vi "Drive Controller.vi"(8 "error in":errorcluster) -> ()   [LabVIEW 2019]
doc: "This VI executes continuously carrying out the current operation and responding to updates or new operation requests. It will often contain the timing or control code that is difficult to place directly in TeleOp. This VI generally opens all sensors and motors and isolates the rest of the robot code from knowing implementation details of how the operations are carried out."
uses:
  <vilib>/Rock Robotics/WPI/Framework/Completion Status.ctl
  Drive Setpoints.ctl
  Drive Operations.ctl
  <vilib>/Rock Robotics/WPI/SafetyOutput/WPI_SafetyOutputConfigMenu.ctl
  <vilib>/Rock Robotics/WPI/RobotDrive/WPI_RobotDriveOpen2MotorWithExistingMotors.vi
panel:
  in  "Radio Buttons":enum32{"Outdoor", "Indoor"}(radio)
  in  "Interactive Values":T1
  in  "Buttons":cluster{"Execute Cmd":bool, "Abort Cmd":bool}
  out "Command Timing":cluster{"Start Time (ms)":u32, "Iterations":i32}
  out "Status":T3
  out "Setpoints":T4(graph)
  out "Current\nCmd":string
  # "Tip: The graph shows the motor setpoints. It may also be helpful to observe inputs and sensor values.\nYou may also want to display tuning or debugging controls."
  # "Interactive Command: You may fill in the settings for a command\nand schedule it with the Execute button. You can observe and abort\nany command while fine tuning the code for the controller."
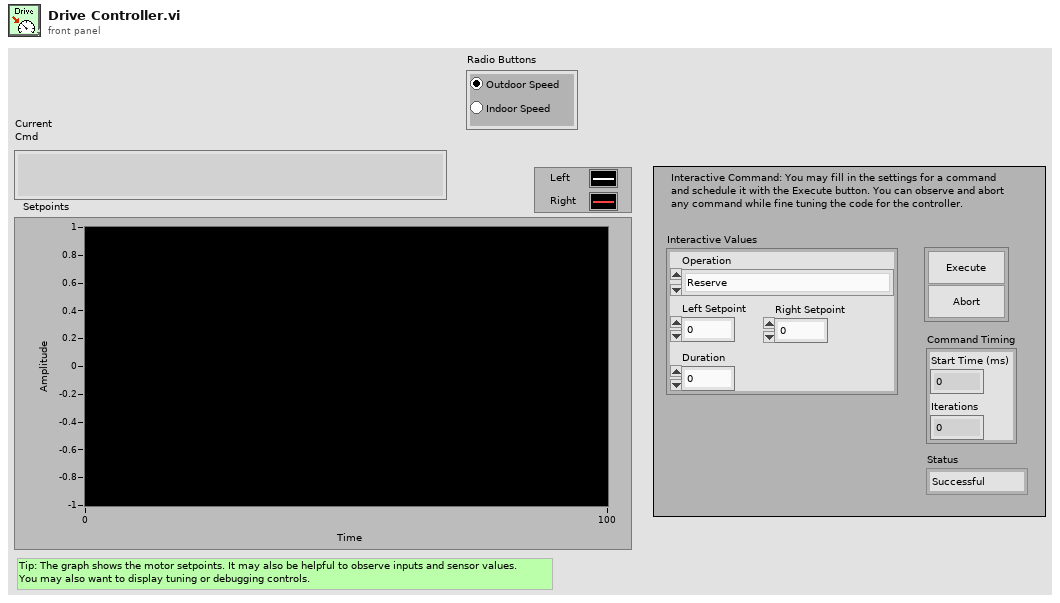
[diagram p1: front panel]
types:
  T1 = typedef "Drive Setpoints.ctl" = cluster{"Operation":T2, "Left Setpoint":dbl, "Right Setpoint":dbl, "Duration":dbl}
  T2 = typedef "Drive Operations.ctl" = enum16{"Reserve", "Read Current", "Immediate", "Drive for Time", "Drive for Distance"}
  T3 = typedef "Completion Status.ctl" = enum16{"Successful", "Aborted", "Incomplete"}
  T4 = cluster{"Left Setpoint":dbl, "Right Setpoint":dbl}
  T5 = enum16{"FollowerType_PercentOutput", "FollowerType_AuxOutput1"}
  T6 = typedef "WPI_SafetyOutputConfigMenu.ctl" = enum16{"Enable", "Disable"}
  T7 = typedef "WPI_MotorControlDeviceRef.ctl" = cluster{"DeviceStatus":errorcluster, "Type":T8, "PWM":cluster{"PWM Channel":T9, "DeadBand":T10}, "CAN":cluster{"Device Number":u8, "SetOutput VI Ref":variant, "GetOutput VI Ref":variant, "Enable VI Ref":variant, "Disable VI Ref":variant, "Data":variant}, "Invert":bool, "DIO PWM":cluster{"PWM \"Enable\" Channel":T9, "DIOChannel":T11, "PWM Rate":dbl}}
  T8 = typedef "WPI_MotorControlType.ctl" = enum16{"PWM", "CAN", "DIO PWM"}
  T9 = typedef "FPGA_DIOPWMChannel.ctl" = enum8{"PWM 0", "PWM 1", "PWM 2", "PWM 3", "PWM 4", "PWM 5", "PWM 6", "PWM 7", "PWM 8", "PWM 9", "PWM MXP 0", "PWM MXP 1", "PWM MXP 2", "PWM MXP 3", "PWM MXP 4", "PWM MXP 5", "PWM MXP 6", "PWM MXP 7", "PWM MXP 8", "PWM MXP 9", "Invalid"}
  T10 = typedef "WPI_PWMDeadband.ctl" = cluster{"Name":string, "maxPositivePwm":i32, "minPositivePwm":i32, "centerPwm":i32, "maxNegativePwm":i32, "minNegativePwm":i32, "angularRange":u16}
  T11 = typedef "FPGA_DIOChannel.ctl" = enum8{"DIO 0", "DIO 1", "DIO 2", "DIO 3", "DIO 4", "DIO 5", "DIO 6", "DIO 7", "DIO 8", "DIO 9", "DIO MXP 0", "DIO MXP 1", "DIO MXP 2", "DIO MXP 3", "DIO MXP 4", "DIO MXP 5", "DIO MXP 6", "DIO MXP 7", "DIO MXP 8", "DIO MXP 9", "DIO MXP 10", "DIO MXP 11", "DIO MXP 12", "DIO MXP 13", "DIO MXP 14", "DIO MXP 15", "SPI Port CS1", "SPI Port CS2", "SPI Port CS3", "SPI Port MISO", "SPI Port MOSI", "Invalid"}
  T12 = typedef "WPI_RobotDriveDevRef.ctl" = cluster{"DevStatus":errorcluster, "Motors[]":T7[], "Square Inputs":bool, "Max Output":dbl}
  T13 = typedef "Command Status Info.ctl" = cluster{"Name":string, "Status":T3, "notifier out":T14}
  T14 = typedef "Completion Notifier.ctl" = refnum<notifier>
  T15 = cluster{"SubSystem Data":T1, cluster{"Start Time (ms)":u32, "Iterations":i32}, cluster{"Command Info":T13, "Description":string, "Default Command":T1, "queue out":refnum<queue>, "Subsystem Name":string}}
  T16 = cluster{"SubSystem Data":T1, cluster{"Start Time (ms)":u32, "Iterations":i32}, "Default Command Arguments":cluster{"Command Info":T13, "Description":string, "Default Command":T1, "queue out":refnum<queue>, "Subsystem Name":string}}
  T17 = cluster{"Don't move motors while reserved":dbl, "Don't move motors while reserved":dbl}
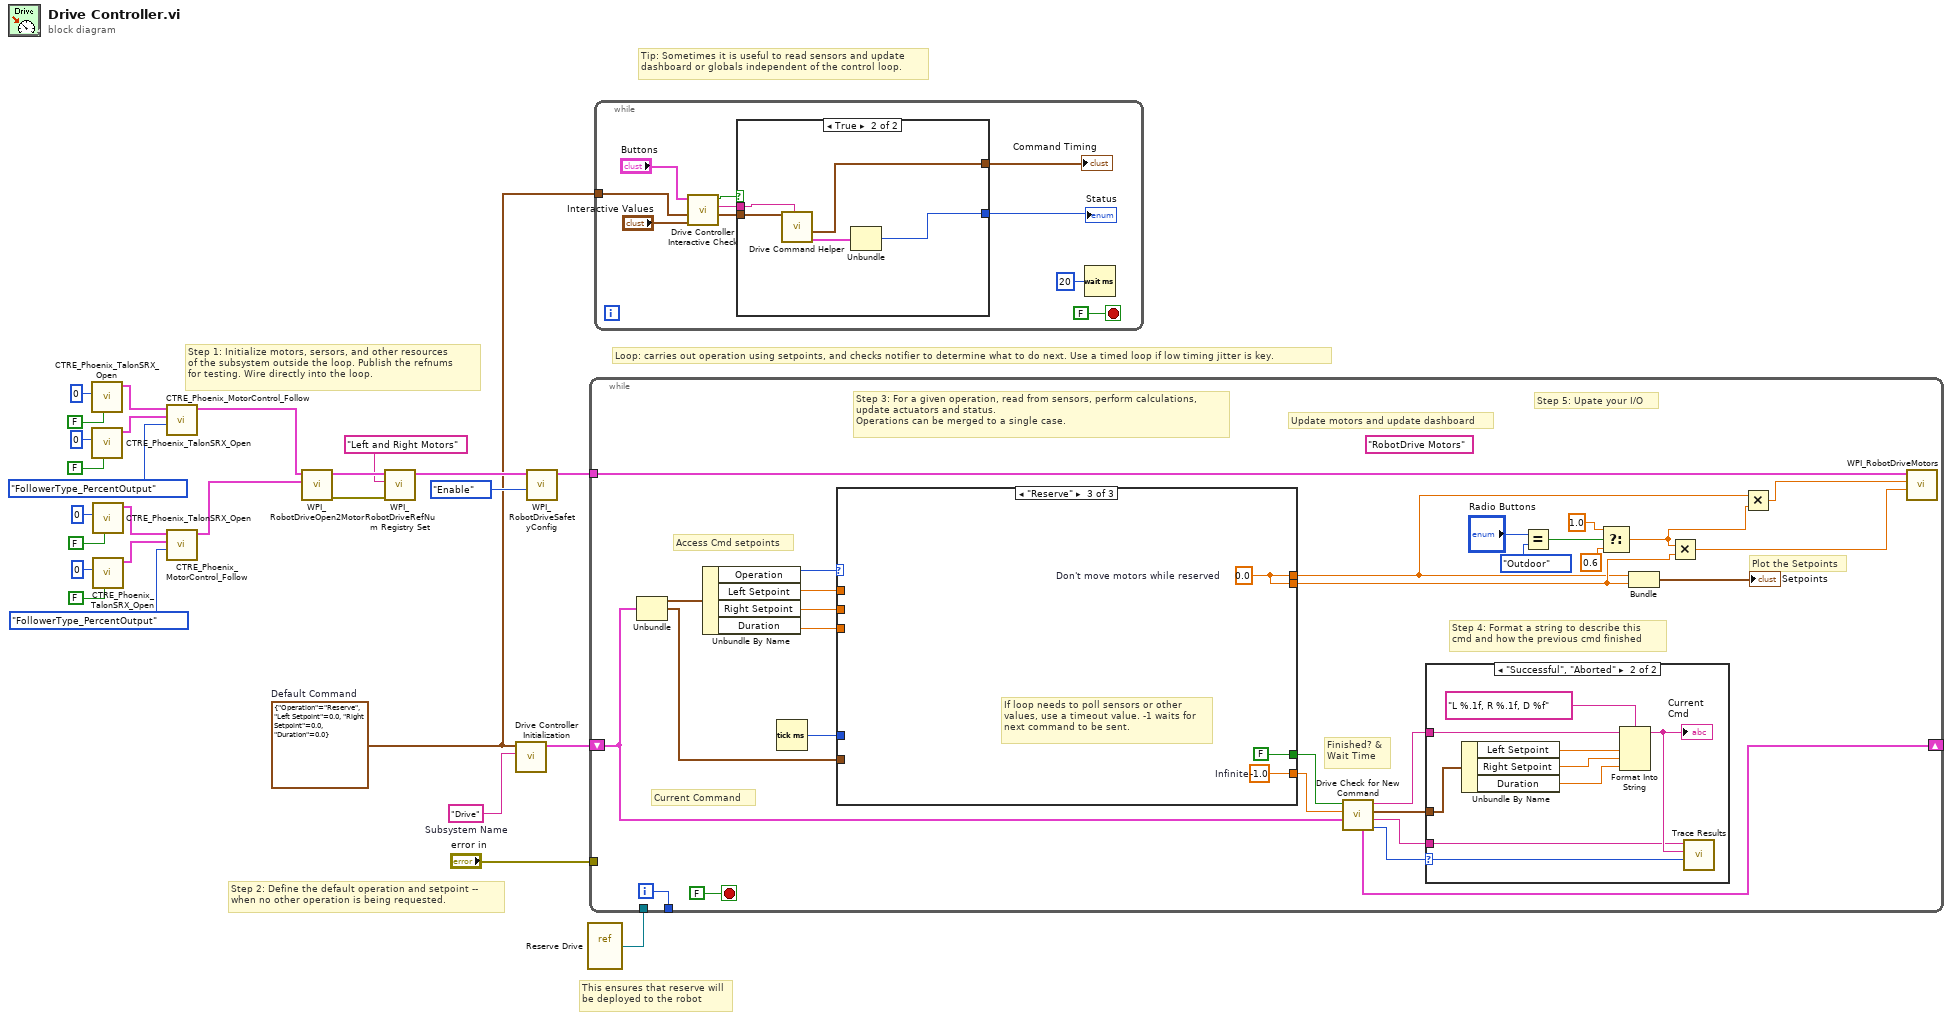
[diagram p0: block diagram]
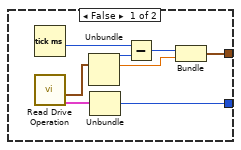
[diagram p2: hidden frame]
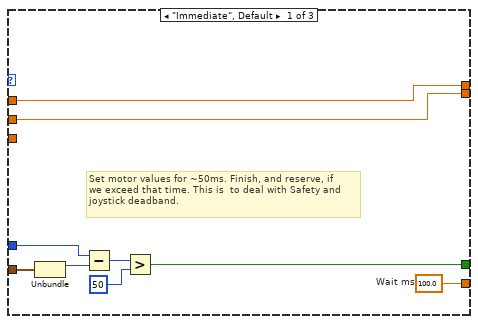
[diagram p4: hidden frame]
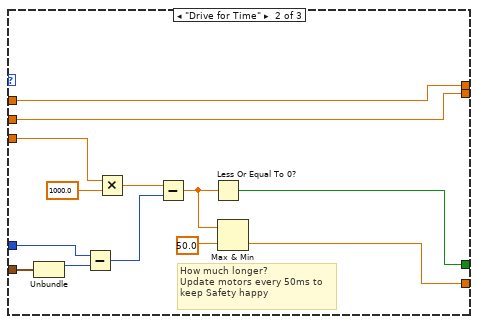
[diagram p5: hidden frame]
diagram:
  w17 = T1 {"Operation"=enum."Reserve", "Left Setpoint"=0.0, "Right Setpoint"=0.0, "Duration"=0.0}  # Default Command
  w27 = "Drive"  # Subsystem Name
  # "This ensures that reserve will\nbe deployed to the robot"
  # "Tip: Sometimes it is useful to read sensors and update\ndashboard or globals independent of the control loop."
  # "Step 2: Define the default operation and setpoint --\nwhen no other operation is being requested."
  # "Step 1: Initialize motors, sersors, and other resources\nof the subsystem outside the loop. Publish the refnums\nfor testing. Wire directly into the loop."
  # "Loop: carries out operation using setpoints, and checks notifier to determine what to do next. Use a timed loop if low timing jitter is key."
  n1 = call <vilib>:"CTRE_Phoenix_TalonSRX_Open.vi"("Invert"=FALSE, "Device Number"=u8 0) -> ("CAN Talon SRX Ref"=w9:T7)  [unwired: 8 in, 1 out]
  n2 = call <vilib>:"CTRE_Phoenix_TalonSRX_Open.vi"("Invert"=FALSE, "Device Number"=u8 0) -> ("CAN Talon SRX Ref"=w8:T7)  [unwired: 8 in, 1 out]
  n3 = call <vilib>:"CTRE_Phoenix_TalonSRX_Open.vi"("Invert"=FALSE, "Device Number"=u8 0) -> ("CAN Talon SRX Ref"=w16:T7)  [unwired: 8 in, 1 out]
  n4 = call <vilib>:"CTRE_Phoenix_TalonSRX_Open.vi"("Invert"=FALSE, "Device Number"=u8 0) -> ("CAN Talon SRX Ref"=w15:T7)  [unwired: 8 in, 1 out]
  n5 = call <vilib>:"CTRE_Phoenix_MotorControl_Follow.vi"("FollowerType"=T5."FollowerType_PercentOutput", "Master Controller to Follow"=w8, "PhoenixMotorControlDevRef"=w9) -> ("PhoenixMotorControlDevRef"=w2:T7)  [unwired: 7 in, 1 out]
  n6 = call <vilib>:"CTRE_Phoenix_MotorControl_Follow.vi"("FollowerType"=T5."FollowerType_PercentOutput", "Master Controller to Follow"=w15, "PhoenixMotorControlDevRef"=w16) -> ("PhoenixMotorControlDevRef"=w1:T7)  [unwired: 7 in, 1 out]
  n7 = call-poly <vilib>:"WPI_RobotDriveOpen2Motor.vi"("Right Motor Dev Ref"=w1, "Left Motor Dev Ref"=w2) -> ("error out"=w24:errorcluster, "RobotDriveDevRef"=w26:T12)  [unwired: 3 in, 5 out]
  n8 = call <vilib>:"WPI_RobotDriveRefNum Registry Set.vi"("error in (no error)"=w24, "refnum name"="Left and Right Motors", "RobotDriveDevRef"=w26) -> ("RobotDriveDevRef"=w23:T12)  [unwired: 1 in, 7 out]
  n9 = call "Drive Controller Initialization.vi"("Subsystem Name"=w27, "Default Command"=w17) -> ("Current Command"=w19:T15)  [unwired: 9 in]
  n10 = call <vilib>:"WPI_RobotDriveSafetyConfig.vi"("mode"=WPI_SafetyOutputConfigMenu."Enable", "RobotDriveDevRef"=w23) -> ("RobotDriveDevRef"=w21:T12)  [unwired: 8 in, 1 out]
  n11 = vi-ref "Reserve Drive.vi"() -> (w18:refnum<vi>)
  n12 = while {
    shift-right: [w45] -> _
    shift-left: w19 -> [w38]
    tunnel: [w55] -> _
    tunnel: w21 -> [w53]
    tunnel: "error in" -> [_]
    tunnel: w18 -> [_]
    i -> [w55]
    stop <- FALSE stop-if-true
    (unwired) "RobotDrive Motors" ("Name")
    # "Step 5: Upate your I/O"
    # "Step 4: Format a string to describe this\ncmd and how the previous cmd finished"
    # "Current Command"
    # "Update motors and update dashboard"
    # "Plot the Setpoints"
    # "Access Cmd setpoints"
    # "Finished? &\nWait Time"
    # "Step 3: For a given operation, read from sensors, perform calculations,\nupdate actuators and status.\nOperations can be merged to a single case."
    n13 = Unbundle(w38) -> ("SubSystem Data"=w52:T1, w39:cluster{"Start Time (ms)":u32, "Iterations":i32})  [unwired: 1 out]
    n14 = Unbundle By Name(w52) -> ("Operation"=w51:T2, "Left Setpoint"=w50:dbl, "Right Setpoint"=w49:dbl, "Duration"=w48:dbl)
    n15 = Tick Count (ms)() -> (millisecond timer value=w47:u32)
    n16 = case shown="\"Reserve\"" w51 {
      tunnel: [w74 w75 w90] -> w44
      tunnel: [w67 w82 FALSE ("ignore previous (F)")] -> w43
      tunnel: w39 -> [w66 w84 _]
      tunnel: [w73 w81 w88] -> w35
      tunnel: [w72 w80 w88] -> w37
      tunnel: w50 -> [w73 w81 _]
      tunnel: w49 -> [w72 w80 _]
      tunnel: w48 -> [_ w79 _]
      tunnel: w47 -> [w68 w78 _]
      frame "Immediate", Default {
        w74 = 100.0  # Wait ms
        # "Set motor values for ~50ms. Finish, and reserve, if\nwe exceed that time. This is  to deal with Safety and\njoystick deadband."
        n17 = Unbundle(w66) -> ("Start Time (ms)"=w69:u32)  [unwired: 1 out]
        n18 = Subtract(x=w68, y=w69) -> (x-y=w70:u32)
        n19 = Greater?(x=w70, y=u8 50 ("Left Motor")) -> (0:w67:bool)
      }
      frame "Drive for Time" {
        # "How much longer?\nUpdate motors every 50ms to\nkeep Safety happy"
        n20 = Unbundle(w84) -> ("Start Time (ms)"=w83:u32)  [unwired: 1 out]
        n21 = Subtract(x=w78, y=w83) -> (x-y=w87:u32)
        n22 = Multiply(x=w79, y=1000.0) -> (x*y=w86:dbl)
        n23 = Subtract(x=w86, y=w87) -> (x-y=w77:dbl)
        n24 = Less Or Equal To 0?(x=w77) -> (x <= 0?=w82:bool)
        n25 = Max & Min(x=w77, y=50.0) -> (min(x,y)=w75:dbl)  [unwired: 1 out]
      }
      frame "Reserve" {
        w88 = 0.0  # Don't move motors while reserved
        w90 = -1.0  # Infinite
        # "If loop needs to poll sensors or other\nvalues, use a timeout value. -1 waits for\nnext command to be sent."
      }
    }
    n26 = call "Drive Check for New Command.vi"("input cluster"=w38, "Wait time (ms)"=w44, "Finished?"=w43) -> ("Completion"=w46:T3, "Subsystem Name"=w40:string, "Current Command"=w41:T1, "Initial Trace String"=w42:string, "Next Command"=w45:T16)  [unwired: 4 in]
    n27 = case shown="\"Successful\", \"Aborted\"" w46 {
      selector: w46 -> [_ w65]
      tunnel: w42 -> [_ w60]
      tunnel: w41 -> [_ w61]
      tunnel: w40 -> [_ w57]
      frame "Incomplete", Default {
        # "Continuing current command"
      }
      frame "Successful", "Aborted" {
        # "Report and setup for next command"
        n28 = Unbundle By Name(w61) -> ("Left Setpoint"=w63:dbl, "Right Setpoint"=w64:dbl, "Duration"=w58:dbl)
        n29 = Format Into String(format string="L %.1f, R %.1f, D %f", initial string=w60, w63, w64, w58) -> (resulting string=w59:string)  [unwired: 1 in, 1 out]
        "Current\nCmd" <- w59
        n30 = call <vilib>:"Trace Results.vi"("Status of previous command"=w65, "Description"=w59, "Subsystem"=w57) -> ()  [unwired: 9 in]
      }
    }
    n31 = Equal?(x="Radio Buttons", y=enum32{"Outdoor", "Indoor"}."Outdoor") -> (x = y?=w30:bool)
    n32 = Select(t=1.0, s=w30, f=0.6) -> (s? t:f=w33:dbl)
    n33 = Bundle("Don't move motors while reserved"=w35, "Don't move motors while reserved"=w37) -> (→"Setpoints":T17)  [unwired: 1 in]
    n34 = Multiply(x=w33, y=w37) -> (x*y=w36:dbl)
    n35 = Multiply(x=w35, y=w33) -> (x*y=w34:dbl)
    n36 = call <vilib>:"WPI_RobotDriveMotors.vi"("RightSpeed"=w36, "LeftSpeed"=w34, "RobotDriveDevRef"=w53) -> ()  [unwired: 1 in, 8 out]
  }
  n37 = while {
    tunnel: w17 -> [w92]
    stop <- FALSE stop-if-true
    n38 = call "Drive Controller Interactive Check.vi"("Interactive Command In"="Interactive Values", "Default Command"=w92, "Buttons"="Buttons") -> ("Interactive Command Out"=w94:T1, "Trace String"=w95:string, "Schedule"=w96:bool)  [unwired: 6 in]
    n39 = case shown="True" w96 {
      tunnel: [w105 w113] -> w97
      tunnel: [w104 w109] -> w98
      tunnel: w95 -> [_ w111]
      tunnel: w94 -> [_ w110]
      frame False {
        n40 = Tick Count (ms)() -> (millisecond timer value=w108:u32)
        n41 = call "Read Drive Operation.vi"() -> ("Command Info"=w102:T13, "SubSystem Data"=w101:T1)  [unwired: 9 in, 1 out]
        n42 = Unbundle(w101) -> ("Operation"=w106:T2, "Left Setpoint"=w103:dbl)  [unwired: 2 out]
        n43 = Unbundle(w102) -> ("Status"=w105:T3)  [unwired: 2 out]
        n44 = Subtract(x=w108, y=w106) -> (x-y=w107:u32)
        n45 = Bundle(w107, "Left Setpoint"=w103) -> (w104:cluster{u32, "Left Setpoint":dbl})  [unwired: 1 in]
      }
      frame True {
        n46 = call "Drive Command Helper.vi"("Description"=w111, "SubSystem Data"=w110) -> ("Command Info Out"=w112:T13, "Command Timing"=w109:cluster{"Start Time (ms)":u32, "Iterations":i32})  [unwired: 7 in, 1 out]
        n47 = Unbundle(w112) -> ("Status"=w113:T3)  [unwired: 2 out]
      }
    }
    "Status" <- w97
    "Command Timing" <- w98
    n48 = Wait (ms)(milliseconds to wait=u32 20) -> ()  [unwired: 1 out]
  }
